vi "flappy--mathstring--load   -- V1.vi"(0 "mathstring IN":string="\"008_040924\" ->   <|  \n\"T\"->  4.0  , \n\"θ\"-> 0 , \n\"vproj\"  -> 0.690,\n\"B\" -> 60 ,\n\"plain\" -> 23\n  |>   , \n  \n    \n\"010_040924\" ->   <|  \n\"T\"->  4.0  , \n\"θ\"-> 30  , \n\"vproj\"  -> 0.600,\n\"B\" -> 60 ,\n\"plain\" -> 23\n  |>   , \n  \n\"011_040924\" ->   <|  \n\"T\"->  4.0  , \n\"θ\"-> 60  , \n\"vproj\"  -> 0.348,\n\"B\" -> 60 ,\n\"plain\" -> 23\n  |>   ,   \n  \n  \n\"002_041024\" ->   <|  \n\"T\"->  4.0  , \n\"θ\"-> 90  , \n\"vproj\"  -> 0.00,\n\"B\" -> 60 ,\n\"plain\" -> 23\n  |>   ,\n   \n    \n\"003_041024\" ->   <|  \n\"T\"->  4.0  , \n\"θ\"-> 120  , \n\"vproj\"  -> -0.340,\n\"B\" -> 60 ,\n\"plain\" -> 23\n  |>   ,\n\n\"004_041024\" ->   <|  \n\"T\"->  4.0  , \n\"θ\"-> 160  , \n\"vproj\"  -> -0.663,\n\"B\" -> 60 ,\n\"plain\" -> 23\n  |>   , \n  \n\"005_041024\" ->   <|  \n\"T\"->  4.0  , \n\"θ\"-> 180  , \n\"vproj\"  -> -0.699,\n\"B\" -> 60 ,\n\"plain\" -> 23\n  |>   , \n  \n\"006_041024\" ->   <|  \n\"T\"->  4.0  , \n\"θ\"-> 165  , \n\"vproj\"  -> -0.677,\n\"B\" -> 60 ,\n\"plain\" -> 23\n  |>   ,\n  \n\"007_041024\" ->   <|  \n\"T\"->  4.0  , \n\"θ\"-> 150  , \n\"vproj\"  -> -0.603,\n\"B\" -> 60 ,\n\"plain\" -> 23\n  |>   ,\n  \n\"008_041024\" ->   <|  \n\"T\"->  4.0  , \n\"θ\"-> 135  , \n\"vproj\"  -> -0.496,\n\"B\" -> 60 ,\n\"plain\" -> 23\n  |>   ,\n  \n\"009_041024\" ->   <|  \n\"T\"->  4.0  , \n\"θ\"-> 105  , \n\"vproj\"  -> -0.178,\n\"B\" -> 60 ,\n\"plain\" -> 23\n  |>   ,\n  \n\"010_041024\" ->   <|  \n\"T\"->  4.0  , \n\"θ\"-> 95  , \n\"vproj\"  -> -0.057,\n\"B\" -> 60 ,\n\"plain\" -> 23\n  |>   ,\n  \n\"011_041024\" ->   <|  \n\"T\"->  4.0  , \n\"θ\"-> 85  , \n\"vproj\"  -> +0.065,\n\"B\" -> 60 ,\n\"plain\" -> 23\n  |>   ,\n  \n\"012_041024\" ->   <|  \n\"T\"->  4.0  , \n\"θ\"-> 75  , \n\"vproj\"  -> +0.183,\n\"B\" -> 60 ,\n\"plain\" -> 23\n  |>   , \n  \n\"013_041024\" ->   <|  \n\"T\"->  4.0  , \n\"θ\"-> 45  , \n\"vproj\"  -> +0.494,\n\"B\" -> 60 ,\n\"plain\" -> 23\n  |>   , \n  \n\"003_041124\" ->   <|  \n\"T\"->  4.0  , \n\"θ\"-> 15  , \n\"vproj\"  -> +0.673,\n\"B\" -> 60 ,\n\"plain\" -> 23\n  |>   ,  \n  \n\"004_041124\" ->   <|  \n\"T\"->  4.0  , \n\"θ\"-> 50  , \n\"vproj\"  -> +0.442,\n\"B\" -> 60 ,\n\"plain\" -> 23\n  |>   ,\n  \n\"005_041124\" ->   <|  \n\"T\"->  4.0  , \n\"θ\"-> 67  , \n\"vproj\"  -> +0.269,\n\"B\" -> 60 ,\n\"plain\" -> 23\n  |>   ,\n  \n\"006_041124\" ->   <|  \n\"T\"->  4.0  , \n\"θ\"-> 55  , \n\"vproj\"  -> +0.397,\n\"B\" -> 60 ,\n\"plain\" -> 23\n  |>   ,   \n  \n\"007_041124\" ->   <|  \n\"T\"->  4.0  , \n\"θ\"-> 112  , \n\"vproj\"  -> -0.260,\n\"B\" -> 60 ,\n\"plain\" -> 23\n  |>   ,  \n  \n\"008_041124\" ->   <|  \n\"T\"->  4.0  , \n\"θ\"-> 128  , \n\"vproj\"  -> -0.432,\n\"B\" -> 60 ,\n\"plain\" -> 23\n  |>   , \n  \n\"009_041124\" ->   <|  \n\"T\"->  4.0  , \n\"θ\"-> 155  , \n\"vproj\"  -> -0.634,\n\"B\" -> 60 ,\n\"plain\" -> 23\n  |>   , \n  \n\"010_041124\" ->   <|  \n\"T\"->  4.0  , \n\"θ\"-> 151  , \n\"vproj\"  -> -0.615,\n\"B\" -> 60 ,\n\"plain\" -> 23\n  |>   ,   \n  \n\"011_041124\" ->   <|  \n\"T\"->  4.0  , \n\"θ\"-> 157  , \n\"vproj\"  -> -0.648,\n\"B\" -> 60 ,\n\"plain\" -> 23\n  |>   ,  \n  \n  \n\"002_041224\" ->   <|  \n\"T\"->  4.0  , \n\"θ\"-> 170  , \n\"vproj\"  -> -0.690,\n\"B\" -> 60 ,\n\"plain\" -> 23\n  |>   ,\n  \n\"003_041224\" ->   <|  \n\"T\"->  4.0  , \n\"θ\"-> 153  , \n\"vproj\"  -> -0.625,\n\"B\" -> 60 ,\n\"plain\" -> 23\n  |>   , \n  \n  \n\"004_041224\" ->   <|  \n\"T\"->  10.0  , \n\"θ\"-> 153  , \n\"vproj\"  -> -0.625,\n\"B\" -> 60 ,\n\"plain\" -> 23\n  |>   ,\n  \n  \n\"005_041224\" ->   <|  \n\"T\"->  20.0  , \n\"θ\"-> 153  , \n\"vproj\"  -> -0.625,\n\"B\" -> 60 ,\n\"plain\" -> 23\n  |>   , \n  \n\"006_041224\" ->   <|  \n\"T\"->  30.0  , \n\"θ\"-> 153  , \n\"vproj\"  -> -0.625,\n\"B\" -> 60 ,\n\"plain\" -> 23\n  |>   ,\n  \n  \n\"007_041224\" ->   <|  \n\"T\"->  25.0  , \n\"θ\"-> 153  , \n\"vproj\"  -> -0.625,\n\"B\" -> 60 ,\n\"plain\" -> 23\n  |>   , \n  \n  \n\"008_041224\" ->   <|  \n\"T\"->  15.0  , \n\"θ\"-> 153  , \n\"vproj\"  -> -0.625,\n\"B\" -> 60 ,\n\"plain\" -> 23\n  |>   , \n  \n  \n\"009_041224\" ->   <|  \n\"T\"->  17.0  , \n\"θ\"-> 153  , \n\"vproj\"  -> -0.625,\n\"B\" -> 60 ,\n\"plain\" -> 23\n  |>   , \n  \n  \n  \n  \n\"004_042224\" ->   <|  \n\"T\"->  4.0  , \n\"θ\"-> 15  , \n\"vproj\"  -> +0.670,\n\"B\" -> 60 ,\n\"plain\" -> 23\n  |>   ,   \n  \n  \n\"005_042224\" ->   <|  \n\"T\"->  4.0  , \n\"θ\"-> 20  , \n\"vproj\"  -> +0.651,\n\"B\" -> 60 ,\n\"plain\" -> 23\n  |>   ,\n  \n\"006_042224\" ->   <|  \n\"T\"->  4.0  , \n\"θ\"-> 25  , \n\"vproj\"  -> +0.628,\n\"B\" -> 60 ,\n\"plain\" -> 23\n  |>   ,\n  \n  \n\"007_042224\" ->   <|  \n\"T\"->  4.0  , \n\"θ\"-> 30  , \n\"vproj\"  -> +0.603,\n\"B\" -> 60 ,\n\"plain\" -> 23\n  |>   , \n  \n\"008_042224\" ->   <|  \n\"T\"->  4.0  , \n\"θ\"-> 40  , \n\"vproj\"  -> +0.533,\n\"B\" -> 60 ,\n\"plain\" -> 23\n  |>   ,\n  \n  \n  \n\"009_042224\" ->   <|  \n\"T\"->  4.0  , \n\"θ\"-> 53  , \n\"vproj\"  -> +0.415,\n\"B\" -> 60 ,\n\"plain\" -> 23\n  |>   , \n  \n  \n\"010_042224\" ->   <|  \n\"T\"->  4.0  , \n\"θ\"-> 65  , \n\"vproj\"  -> +0.288,\n\"B\" -> 60 ,\n\"plain\" -> 23\n  |>   ,   \n  \n  \n\"011_042224\" ->   <|  \n\"T\"->  4.0  , \n\"θ\"-> 160  , \n\"vproj\"  -> -0.661,\n\"B\" -> 60 ,\n\"plain\" -> 23\n  |>   ,  \n  \n  \n\"013_042224\" ->   <|  \n\"T\"->  4.0  , \n\"θ\"-> 163  , \n\"vproj\"  -> -0.674,\n\"B\" -> 60 ,\n\"plain\" -> 23\n  |>   ,                                                               \n                                              ", 2 "MAIN folder":path=path "/Users/arkadyshekhter/Library/CloudStorage/Dropbox/shared_KimValBra/UTe2--Apr2024", 9 "data file parameters map":map{T2, T3}(c390), 11 "what? IN":T1={"ignore set of !"=TRUE, "set (1T|2B)"=0, "ignore θ !"=FALSE, "ignore B !"=FALSE, "T (K)"=1.0, "ignore T !"=TRUE, "θ (∘)"=0.0, "B (T)"=0.0, "lookup"={"set of lookup"={0=1.0, 1=2.0}, "all set of"={1.0, 2.0}, "T lookup"={0=0.12, 1=0.122, 2=0.14, 3=0.148, 4=0.15, 5=0.157, 6=0.16, 7=0.168, 8=0.17, 9=0.178, 10=0.179, 11=0.18, 12=0.19, 13=0.197, 14=0.2, 15=0.249, 16=0.25, 17=0.255, 18=0.26, 19=0.3, 20=0.307, 21=0.308, 22=0.31, 23=0.36, 24=0.42, 25=0.43, 26=0.438, 27=0.512, 28=0.52, 29=0.53, 30=0.61, 31=0.62, 32=0.63, 33=0.677, 34=0.81, 35=0.82, 36=0.83, 37=1.0, 38=1.1, 39=1.12, 40=1.13, 41=1.25, 42=1.28, 43=1.31, 44=1.39, 45=1.5, 46=1.52, 47=1.55, 48=1.6, 49=1.7, 50=1.8, 51=1.9, 52=2.1, 53=2.3, 54=3.0, 55=3.07, 56=3.1, 57=3.11, 58=5.5, 59=5.7, 60=5.75}, "θ lookup"={0=0.0, 1=30.0, 2=45.0, 3=60.0, 4=90.0}, "B lookup"={0=0.0, 1=1.0, 2=2.0, 3=4.0, 4=5.0, 5=6.0, 6=7.0, 7=8.0, 8=9.0, 9=10.0, 10=11.0, 11=12.0}, "all T's"={0.12, 0.122, 0.14, 0.148, 0.15, 0.157, 0.16, 0.168, 0.17, 0.178, 0.179, 0.18, 0.19, 0.197, 0.2, 0.249, 0.25, 0.255, 0.26, 0.3, 0.307, 0.308, 0.31, 0.36, 0.42, 0.43, 0.438, 0.512, 0.52, 0.53, 0.61, 0.62, 0.63, 0.677, 0.81, 0.82, 0.83, 1.0, 1.1, 1.12, 1.13, 1.25, 1.28, 1.31, 1.39, 1.5, 1.52, 1.55, 1.6, 1.7, 1.8, 1.9, 2.1, 2.3, 3.0, 3.07, 3.1, 3.11, 5.5, 5.7, 5.75}, "all θ's"={0.0, 30.0, 45.0, 60.0, 90.0}, "all B's"={0.0, 1.0, 2.0, 4.0, 5.0, 6.0, 7.0, 8.0, 9.0, 10.0, 11.0, 12.0}, "all sides"={4000.0, 8000.0}, "side lookup"={0=4000.0, 1=8000.0}}} {"B (T)" items=["0.000", "1.000", "2.000", "4.000", "5.000", "6.000", "7.000", "8.000", "9.000", "10.000", "11.000", "12.000"]; "θ (∘)" items=["0.000", "30.000", "45.000", "60.000", "90.000"]; "T (K)" items=["0.120", "0.122", "0.140", "0.148", "0.150", "0.157", "0.160", "0.168", "0.170", "0.178", "0.179", "0.180", "0.190", "0.197", "0.200", "0.249", "0.250", "0.255", "0.260", "0.300", "0.307", "0.308", "0.310", "0.360", "0.420", "0.430", "0.438", "0.512", "0.520", "0.530", "0.610", "0.620", "0.630", "0.677", "0.810", "0.820", "0.830", "1.000", "1.100", "1.120", "1.130", "1.250", "1.280", "1.310", "1.390", "1.500", "1.520", "1.550", "1.600", "1.700", "1.800", "1.900", "2.100", "2.300", "3.000", "3.070", "3.100", "3.110", "5.500", "5.700", "5.750"]; "set (1T|2B)" items=["1", "2"]}, 13 "data file pattern":string="p_c3_*.tdms") -> (4 "all short filenames":map{string, string}(c390), 6 "temps&degs":map{string, map{T2, dbl}}(c390), 8 "mathematica thing":map{string, map{T2, dbl}}(c390)={"002_041024"={enum."ζ"=0.0, enum."τ1"=0.0, enum."τS"=0.0, enum."τN"=0.0, enum."τC"=0.0, enum."κ0"=0.0, enum."m1"=0.0, enum."m2"=0.0, enum."m3"=0.0, enum."T (K)"=4.0, enum."B (T)"=60.0, enum."θ (deg)"=90.0, enum."Re(offset)"=0.0, enum."Im(offset)"=0.0, enum."στ1"=0.0, enum."στS"=0.0, enum."στN"=0.0, enum."τ11"=0.0, enum."τ12"=0.0, enum."τ22"=0.0, enum."τN1"=0.0, enum."τN2"=0.0, enum."σηlogτ1"=0.0, enum."σηlogτS"=0.0, enum."σηlogτN"=0.0, enum."σlogτ1"=0.0, enum."σlogτS"=0.0, enum."σlogτN"=0.0, enum."σητ1"=0.0, enum."σητS"=0.0, enum."σητN"=0.0, enum."noiseT"=0.0, enum."plain"=23.0, enum."vproj"=0.0}, "002_041224"={enum."ζ"=0.0, enum."τ1"=0.0, enum."τS"=0.0, enum."τN"=0.0, enum."τC"=0.0, enum."κ0"=0.0, enum."m1"=0.0, enum."m2"=0.0, enum."m3"=0.0, enum."T (K)"=4.0, enum."B (T)"=60.0, enum."θ (deg)"=170.0, enum."Re(offset)"=0.0, enum."Im(offset)"=0.0, enum."στ1"=0.0, enum."στS"=0.0, enum."στN"=0.0, enum."τ11"=0.0, enum."τ12"=0.0, enum."τ22"=0.0, enum."τN1"=0.0, enum."τN2"=0.0, enum."σηlogτ1"=0.0, enum."σηlogτS"=0.0, enum."σηlogτN"=0.0, enum."σlogτ1"=0.0, enum."σlogτS"=0.0, enum."σlogτN"=0.0, enum."σητ1"=0.0, enum."σητS"=0.0, enum."σητN"=0.0, enum."noiseT"=0.0, enum."plain"=23.0, enum."vproj"=-0.69}, "003_041024"={enum."ζ"=0.0, enum."τ1"=0.0, enum."τS"=0.0, enum."τN"=0.0, enum."τC"=0.0, enum."κ0"=0.0, enum."m1"=0.0, enum."m2"=0.0, enum."m3"=0.0, enum."T (K)"=4.0, enum."B (T)"=60.0, enum."θ (deg)"=120.0, enum."Re(offset)"=0.0, enum."Im(offset)"=0.0, enum."στ1"=0.0, enum."στS"=0.0, enum."στN"=0.0, enum."τ11"=0.0, enum."τ12"=0.0, enum."τ22"=0.0, enum."τN1"=0.0, enum."τN2"=0.0, enum."σηlogτ1"=0.0, enum."σηlogτS"=0.0, enum."σηlogτN"=0.0, enum."σlogτ1"=0.0, enum."σlogτS"=0.0, enum."σlogτN"=0.0, enum."σητ1"=0.0, enum."σητS"=0.0, enum."σητN"=0.0, enum."noiseT"=0.0, enum."plain"=23.0, enum."vproj"=-0.34}, "003_041124"={enum."ζ"=0.0, enum."τ1"=0.0, enum."τS"=0.0, enum."τN"=0.0, enum."τC"=0.0, enum."κ0"=0.0, enum."m1"=0.0, enum."m2"=0.0, enum."m3"=0.0, enum."T (K)"=4.0, enum."B (T)"=60.0, enum."θ (deg)"=15.0, enum."Re(offset)"=0.0, enum."Im(offset)"=0.0, enum."στ1"=0.0, enum."στS"=0.0, enum."στN"=0.0, enum."τ11"=0.0, enum."τ12"=0.0, enum."τ22"=0.0, enum."τN1"=0.0, enum."τN2"=0.0, enum."σηlogτ1"=0.0, enum."σηlogτS"=0.0, enum."σηlogτN"=0.0, enum."σlogτ1"=0.0, enum."σlogτS"=0.0, enum."σlogτN"=0.0, enum."σητ1"=0.0, enum."σητS"=0.0, enum."σητN"=0.0, enum."noiseT"=0.0, enum."plain"=23.0, enum."vproj"=0.673}, "003_041224"={enum."ζ"=0.0, enum."τ1"=0.0, enum."τS"=0.0, enum."τN"=0.0, enum."τC"=0.0, enum."κ0"=0.0, enum."m1"=0.0, enum."m2"=0.0, enum."m3"=0.0, enum."T (K)"=4.0, enum."B (T)"=60.0, enum."θ (deg)"=153.0, enum."Re(offset)"=0.0, enum."Im(offset)"=0.0, enum."στ1"=0.0, enum."στS"=0.0, enum."στN"=0.0, enum."τ11"=0.0, enum."τ12"=0.0, enum."τ22"=0.0, enum."τN1"=0.0, enum."τN2"=0.0, enum."σηlogτ1"=0.0, enum."σηlogτS"=0.0, enum."σηlogτN"=0.0, enum."σlogτ1"=0.0, enum."σlogτS"=0.0, enum."σlogτN"=0.0, enum."σητ1"=0.0, enum."σητS"=0.0, enum."σητN"=0.0, enum."noiseT"=0.0, enum."plain"=23.0, enum."vproj"=-0.625}, "004_041024"={enum."ζ"=0.0, enum."τ1"=0.0, enum."τS"=0.0, enum."τN"=0.0, enum."τC"=0.0, enum."κ0"=0.0, enum."m1"=0.0, enum."m2"=0.0, enum."m3"=0.0, enum."T (K)"=4.0, enum."B (T)"=60.0, enum."θ (deg)"=160.0, enum."Re(offset)"=0.0, enum."Im(offset)"=0.0, enum."στ1"=0.0, enum."στS"=0.0, enum."στN"=0.0, enum."τ11"=0.0, enum."τ12"=0.0, enum."τ22"=0.0, enum."τN1"=0.0, enum."τN2"=0.0, enum."σηlogτ1"=0.0, enum."σηlogτS"=0.0, enum."σηlogτN"=0.0, enum."σlogτ1"=0.0, enum."σlogτS"=0.0, enum."σlogτN"=0.0, enum."σητ1"=0.0, enum."σητS"=0.0, enum."σητN"=0.0, enum."noiseT"=0.0, enum."plain"=23.0, enum."vproj"=-0.663}, "004_041124"={enum."ζ"=0.0, enum."τ1"=0.0, enum."τS"=0.0, enum."τN"=0.0, enum."τC"=0.0, enum."κ0"=0.0, enum."m1"=0.0, enum."m2"=0.0, enum."m3"=0.0, enum."T (K)"=4.0, enum."B (T)"=60.0, enum."θ (deg)"=50.0, enum."Re(offset)"=0.0, enum."Im(offset)"=0.0, enum."στ1"=0.0, enum."στS"=0.0, enum."στN"=0.0, enum."τ11"=0.0, enum."τ12"=0.0, enum."τ22"=0.0, enum."τN1"=0.0, enum."τN2"=0.0, enum."σηlogτ1"=0.0, enum."σηlogτS"=0.0, enum."σηlogτN"=0.0, enum."σlogτ1"=0.0, enum."σlogτS"=0.0, enum."σlogτN"=0.0, enum."σητ1"=0.0, enum."σητS"=0.0, enum."σητN"=0.0, enum."noiseT"=0.0, enum."plain"=23.0, enum."vproj"=0.442}, "004_041224"={enum."ζ"=0.0, enum."τ1"=0.0, enum."τS"=0.0, enum."τN"=0.0, enum."τC"=0.0, enum."κ0"=0.0, enum."m1"=0.0, enum."m2"=0.0, enum."m3"=0.0, enum."T (K)"=10.0, enum."B (T)"=60.0, enum."θ (deg)"=153.0, enum."Re(offset)"=0.0, enum."Im(offset)"=0.0, enum."στ1"=0.0, enum."στS"=0.0, enum."στN"=0.0, enum."τ11"=0.0, enum."τ12"=0.0, enum."τ22"=0.0, enum."τN1"=0.0, enum."τN2"=0.0, enum."σηlogτ1"=0.0, enum."σηlogτS"=0.0, enum."σηlogτN"=0.0, enum."σlogτ1"=0.0, enum."σlogτS"=0.0, enum."σlogτN"=0.0, enum."σητ1"=0.0, enum."σητS"=0.0, enum."σητN"=0.0, enum."noiseT"=0.0, enum."plain"=23.0, enum."vproj"=-0.625}, "004_042224"={enum."ζ"=0.0, enum."τ1"=0.0, enum."τS"=0.0, enum."τN"=0.0, enum."τC"=0.0, enum."κ0"=0.0, enum."m1"=0.0, enum."m2"=0.0, enum."m3"=0.0, enum."T (K)"=4.0, enum."B (T)"=60.0, enum."θ (deg)"=15.0, enum."Re(offset)"=0.0, enum."Im(offset)"=0.0, enum."στ1"=0.0, enum."στS"=0.0, enum."στN"=0.0, enum."τ11"=0.0, enum."τ12"=0.0, enum."τ22"=0.0, enum."τN1"=0.0, enum."τN2"=0.0, enum."σηlogτ1"=0.0, enum."σηlogτS"=0.0, enum."σηlogτN"=0.0, enum."σlogτ1"=0.0, enum."σlogτS"=0.0, enum."σlogτN"=0.0, enum."σητ1"=0.0, enum."σητS"=0.0, enum."σητN"=0.0, enum."noiseT"=0.0, enum."plain"=23.0, enum."vproj"=0.67}, "005_041024"={enum."ζ"=0.0, enum."τ1"=0.0, enum."τS"=0.0, enum."τN"=0.0, enum."τC"=0.0, enum."κ0"=0.0, enum."m1"=0.0, enum."m2"=0.0, enum."m3"=0.0, enum."T (K)"=4.0, enum."B (T)"=60.0, enum."θ (deg)"=180.0, enum."Re(offset)"=0.0, enum."Im(offset)"=0.0, enum."στ1"=0.0, enum."στS"=0.0, enum."στN"=0.0, enum."τ11"=0.0, enum."τ12"=0.0, enum."τ22"=0.0, enum."τN1"=0.0, enum."τN2"=0.0, enum."σηlogτ1"=0.0, enum."σηlogτS"=0.0, enum."σηlogτN"=0.0, enum."σlogτ1"=0.0, enum."σlogτS"=0.0, enum."σlogτN"=0.0, enum."σητ1"=0.0, enum."σητS"=0.0, enum."σητN"=0.0, enum."noiseT"=0.0, enum."plain"=23.0, enum."vproj"=-0.699}, "005_041124"={enum."ζ"=0.0, enum."τ1"=0.0, enum."τS"=0.0, enum."τN"=0.0, enum."τC"=0.0, enum."κ0"=0.0, enum."m1"=0.0, enum."m2"=0.0, enum."m3"=0.0, enum."T (K)"=4.0, enum."B (T)"=60.0, enum."θ (deg)"=67.0, enum."Re(offset)"=0.0, enum."Im(offset)"=0.0, enum."στ1"=0.0, enum."στS"=0.0, enum."στN"=0.0, enum."τ11"=0.0, enum."τ12"=0.0, enum."τ22"=0.0, enum."τN1"=0.0, enum."τN2"=0.0, enum."σηlogτ1"=0.0, enum."σηlogτS"=0.0, enum."σηlogτN"=0.0, enum."σlogτ1"=0.0, enum."σlogτS"=0.0, enum."σlogτN"=0.0, enum."σητ1"=0.0, enum."σητS"=0.0, enum."σητN"=0.0, enum."noiseT"=0.0, enum."plain"=23.0, enum."vproj"=0.269}, "005_041224"={enum."ζ"=0.0, enum."τ1"=0.0, enum."τS"=0.0, enum."τN"=0.0, enum."τC"=0.0, enum."κ0"=0.0, enum."m1"=0.0, enum."m2"=0.0, enum."m3"=0.0, enum."T (K)"=20.0, enum."B (T)"=60.0, enum."θ (deg)"=153.0, enum."Re(offset)"=0.0, enum."Im(offset)"=0.0, enum."στ1"=0.0, enum."στS"=0.0, enum."στN"=0.0, enum."τ11"=0.0, enum."τ12"=0.0, enum."τ22"=0.0, enum."τN1"=0.0, enum."τN2"=0.0, enum."σηlogτ1"=0.0, enum."σηlogτS"=0.0, enum."σηlogτN"=0.0, enum."σlogτ1"=0.0, enum."σlogτS"=0.0, enum."σlogτN"=0.0, enum."σητ1"=0.0, enum."σητS"=0.0, enum."σητN"=0.0, enum."noiseT"=0.0, enum."plain"=23.0, enum."vproj"=-0.625}, "005_042224"={enum."ζ"=0.0, enum."τ1"=0.0, enum."τS"=0.0, enum."τN"=0.0, enum."τC"=0.0, enum."κ0"=0.0, enum."m1"=0.0, enum."m2"=0.0, enum."m3"=0.0, enum."T (K)"=4.0, enum."B (T)"=60.0, enum."θ (deg)"=20.0, enum."Re(offset)"=0.0, enum."Im(offset)"=0.0, enum."στ1"=0.0, enum."στS"=0.0, enum."στN"=0.0, enum."τ11"=0.0, enum."τ12"=0.0, enum."τ22"=0.0, enum."τN1"=0.0, enum."τN2"=0.0, enum."σηlogτ1"=0.0, enum."σηlogτS"=0.0, enum."σηlogτN"=0.0, enum."σlogτ1"=0.0, enum."σlogτS"=0.0, enum."σlogτN"=0.0, enum."σητ1"=0.0, enum."σητS"=0.0, enum."σητN"=0.0, enum."noiseT"=0.0, enum."plain"=23.0, enum."vproj"=0.651}, "006_041024"={enum."ζ"=0.0, enum."τ1"=0.0, enum."τS"=0.0, enum."τN"=0.0, enum."τC"=0.0, enum."κ0"=0.0, enum."m1"=0.0, enum."m2"=0.0, enum."m3"=0.0, enum."T (K)"=4.0, enum."B (T)"=60.0, enum."θ (deg)"=165.0, enum."Re(offset)"=0.0, enum."Im(offset)"=0.0, enum."στ1"=0.0, enum."στS"=0.0, enum."στN"=0.0, enum."τ11"=0.0, enum."τ12"=0.0, enum."τ22"=0.0, enum."τN1"=0.0, enum."τN2"=0.0, enum."σηlogτ1"=0.0, enum."σηlogτS"=0.0, enum."σηlogτN"=0.0, enum."σlogτ1"=0.0, enum."σlogτS"=0.0, enum."σlogτN"=0.0, enum."σητ1"=0.0, enum."σητS"=0.0, enum."σητN"=0.0, enum."noiseT"=0.0, enum."plain"=23.0, enum."vproj"=-0.677}, "006_041124"={enum."ζ"=0.0, enum."τ1"=0.0, enum."τS"=0.0, enum."τN"=0.0, enum."τC"=0.0, enum."κ0"=0.0, enum."m1"=0.0, enum."m2"=0.0, enum."m3"=0.0, enum."T (K)"=4.0, enum."B (T)"=60.0, enum."θ (deg)"=55.0, enum."Re(offset)"=0.0, enum."Im(offset)"=0.0, enum."στ1"=0.0, enum."στS"=0.0, enum."στN"=0.0, enum."τ11"=0.0, enum."τ12"=0.0, enum."τ22"=0.0, enum."τN1"=0.0, enum."τN2"=0.0, enum."σηlogτ1"=0.0, enum."σηlogτS"=0.0, enum."σηlogτN"=0.0, enum."σlogτ1"=0.0, enum."σlogτS"=0.0, enum."σlogτN"=0.0, enum."σητ1"=0.0, enum."σητS"=0.0, enum."σητN"=0.0, enum."noiseT"=0.0, enum."plain"=23.0, enum."vproj"=0.397}, "006_041224"={enum."ζ"=0.0, enum."τ1"=0.0, enum."τS"=0.0, enum."τN"=0.0, enum."τC"=0.0, enum."κ0"=0.0, enum."m1"=0.0, enum."m2"=0.0, enum."m3"=0.0, enum."T (K)"=30.0, enum."B (T)"=60.0, enum."θ (deg)"=153.0, enum."Re(offset)"=0.0, enum."Im(offset)"=0.0, enum."στ1"=0.0, enum."στS"=0.0, enum."στN"=0.0, enum."τ11"=0.0, enum."τ12"=0.0, enum."τ22"=0.0, enum."τN1"=0.0, enum."τN2"=0.0, enum."σηlogτ1"=0.0, enum."σηlogτS"=0.0, enum."σηlogτN"=0.0, enum."σlogτ1"=0.0, enum."σlogτS"=0.0, enum."σlogτN"=0.0, enum."σητ1"=0.0, enum."σητS"=0.0, enum."σητN"=0.0, enum."noiseT"=0.0, enum."plain"=23.0, enum."vproj"=-0.625}, "006_042224"={enum."ζ"=0.0, enum."τ1"=0.0, enum."τS"=0.0, enum."τN"=0.0, enum."τC"=0.0, enum."κ0"=0.0, enum."m1"=0.0, enum."m2"=0.0, enum."m3"=0.0, enum."T (K)"=4.0, enum."B (T)"=60.0, enum."θ (deg)"=25.0, enum."Re(offset)"=0.0, enum."Im(offset)"=0.0, enum."στ1"=0.0, enum."στS"=0.0, enum."στN"=0.0, enum."τ11"=0.0, enum."τ12"=0.0, enum."τ22"=0.0, enum."τN1"=0.0, enum."τN2"=0.0, enum."σηlogτ1"=0.0, enum."σηlogτS"=0.0, enum."σηlogτN"=0.0, enum."σlogτ1"=0.0, enum."σlogτS"=0.0, enum."σlogτN"=0.0, enum."σητ1"=0.0, enum."σητS"=0.0, enum."σητN"=0.0, enum."noiseT"=0.0, enum."plain"=23.0, enum."vproj"=0.628}, "007_041024"={enum."ζ"=0.0, enum."τ1"=0.0, enum."τS"=0.0, enum."τN"=0.0, enum."τC"=0.0, enum."κ0"=0.0, enum."m1"=0.0, enum."m2"=0.0, enum."m3"=0.0, enum."T (K)"=4.0, enum."B (T)"=60.0, enum."θ (deg)"=150.0, enum."Re(offset)"=0.0, enum."Im(offset)"=0.0, enum."στ1"=0.0, enum."στS"=0.0, enum."στN"=0.0, enum."τ11"=0.0, enum."τ12"=0.0, enum."τ22"=0.0, enum."τN1"=0.0, enum."τN2"=0.0, enum."σηlogτ1"=0.0, enum."σηlogτS"=0.0, enum."σηlogτN"=0.0, enum."σlogτ1"=0.0, enum."σlogτS"=0.0, enum."σlogτN"=0.0, enum."σητ1"=0.0, enum."σητS"=0.0, enum."σητN"=0.0, enum."noiseT"=0.0, enum."plain"=23.0, enum."vproj"=-0.603}, "007_041124"={enum."ζ"=0.0, enum."τ1"=0.0, enum."τS"=0.0, enum."τN"=0.0, enum."τC"=0.0, enum."κ0"=0.0, enum."m1"=0.0, enum."m2"=0.0, enum."m3"=0.0, enum."T (K)"=4.0, enum."B (T)"=60.0, enum."θ (deg)"=112.0, enum."Re(offset)"=0.0, enum."Im(offset)"=0.0, enum."στ1"=0.0, enum."στS"=0.0, enum."στN"=0.0, enum."τ11"=0.0, enum."τ12"=0.0, enum."τ22"=0.0, enum."τN1"=0.0, enum."τN2"=0.0, enum."σηlogτ1"=0.0, enum."σηlogτS"=0.0, enum."σηlogτN"=0.0, enum."σlogτ1"=0.0, enum."σlogτS"=0.0, enum."σlogτN"=0.0, enum."σητ1"=0.0, enum."σητS"=0.0, enum."σητN"=0.0, enum."noiseT"=0.0, enum."plain"=23.0, enum."vproj"=-0.26}, "007_041224"={enum."ζ"=0.0, enum."τ1"=0.0, enum."τS"=0.0, enum."τN"=0.0, enum."τC"=0.0, enum."κ0"=0.0, enum."m1"=0.0, enum."m2"=0.0, enum."m3"=0.0, enum."T (K)"=25.0, enum."B (T)"=60.0, enum."θ (deg)"=153.0, enum."Re(offset)"=0.0, enum."Im(offset)"=0.0, enum."στ1"=0.0, enum."στS"=0.0, enum."στN"=0.0, enum."τ11"=0.0, enum."τ12"=0.0, enum."τ22"=0.0, enum."τN1"=0.0, enum."τN2"=0.0, enum."σηlogτ1"=0.0, enum."σηlogτS"=0.0, enum."σηlogτN"=0.0, enum."σlogτ1"=0.0, enum."σlogτS"=0.0, enum."σlogτN"=0.0, enum."σητ1"=0.0, enum."σητS"=0.0, enum."σητN"=0.0, enum."noiseT"=0.0, enum."plain"=23.0, enum."vproj"=-0.625}, "007_042224"={enum."ζ"=0.0, enum."τ1"=0.0, enum."τS"=0.0, enum."τN"=0.0, enum."τC"=0.0, enum."κ0"=0.0, enum."m1"=0.0, enum."m2"=0.0, enum."m3"=0.0, enum."T (K)"=4.0, enum."B (T)"=60.0, enum."θ (deg)"=30.0, enum."Re(offset)"=0.0, enum."Im(offset)"=0.0, enum."στ1"=0.0, enum."στS"=0.0, enum."στN"=0.0, enum."τ11"=0.0, enum."τ12"=0.0, enum."τ22"=0.0, enum."τN1"=0.0, enum."τN2"=0.0, enum."σηlogτ1"=0.0, enum."σηlogτS"=0.0, enum."σηlogτN"=0.0, enum."σlogτ1"=0.0, enum."σlogτS"=0.0, enum."σlogτN"=0.0, enum."σητ1"=0.0, enum."σητS"=0.0, enum."σητN"=0.0, enum."noiseT"=0.0, enum."plain"=23.0, enum."vproj"=0.603}, "008_040924"={enum."ζ"=0.0, enum."τ1"=0.0, enum."τS"=0.0, enum."τN"=0.0, enum."τC"=0.0, enum."κ0"=0.0, enum."m1"=0.0, enum."m2"=0.0, enum."m3"=0.0, enum."T (K)"=4.0, enum."B (T)"=60.0, enum."θ (deg)"=0.0, enum."Re(offset)"=0.0, enum."Im(offset)"=0.0, enum."στ1"=0.0, enum."στS"=0.0, enum."στN"=0.0, enum."τ11"=0.0, enum."τ12"=0.0, enum."τ22"=0.0, enum."τN1"=0.0, enum."τN2"=0.0, enum."σηlogτ1"=0.0, enum."σηlogτS"=0.0, enum."σηlogτN"=0.0, enum."σlogτ1"=0.0, enum."σlogτS"=0.0, enum."σlogτN"=0.0, enum."σητ1"=0.0, enum."σητS"=0.0, enum."σητN"=0.0, enum."noiseT"=0.0, enum."plain"=23.0, enum."vproj"=0.69}, "008_041024"={enum."ζ"=0.0, enum."τ1"=0.0, enum."τS"=0.0, enum."τN"=0.0, enum."τC"=0.0, enum."κ0"=0.0, enum."m1"=0.0, enum."m2"=0.0, enum."m3"=0.0, enum."T (K)"=4.0, enum."B (T)"=60.0, enum."θ (deg)"=135.0, enum."Re(offset)"=0.0, enum."Im(offset)"=0.0, enum."στ1"=0.0, enum."στS"=0.0, enum."στN"=0.0, enum."τ11"=0.0, enum."τ12"=0.0, enum."τ22"=0.0, enum."τN1"=0.0, enum."τN2"=0.0, enum."σηlogτ1"=0.0, enum."σηlogτS"=0.0, enum."σηlogτN"=0.0, enum."σlogτ1"=0.0, enum."σlogτS"=0.0, enum."σlogτN"=0.0, enum."σητ1"=0.0, enum."σητS"=0.0, enum."σητN"=0.0, enum."noiseT"=0.0, enum."plain"=23.0, enum."vproj"=-0.496}, "008_041124"={enum."ζ"=0.0, enum."τ1"=0.0, enum."τS"=0.0, enum."τN"=0.0, enum."τC"=0.0, enum."κ0"=0.0, enum."m1"=0.0, enum."m2"=0.0, enum."m3"=0.0, enum."T (K)"=4.0, enum."B (T)"=60.0, enum."θ (deg)"=128.0, enum."Re(offset)"=0.0, enum."Im(offset)"=0.0, enum."στ1"=0.0, enum."στS"=0.0, enum."στN"=0.0, enum."τ11"=0.0, enum."τ12"=0.0, enum."τ22"=0.0, enum."τN1"=0.0, enum."τN2"=0.0, enum."σηlogτ1"=0.0, enum."σηlogτS"=0.0, enum."σηlogτN"=0.0, enum."σlogτ1"=0.0, enum."σlogτS"=0.0, enum."σlogτN"=0.0, enum."σητ1"=0.0, enum."σητS"=0.0, enum."σητN"=0.0, enum."noiseT"=0.0, enum."plain"=23.0, enum."vproj"=-0.432}, "008_041224"={enum."ζ"=0.0, enum."τ1"=0.0, enum."τS"=0.0, enum."τN"=0.0, enum."τC"=0.0, enum."κ0"=0.0, enum."m1"=0.0, enum."m2"=0.0, enum."m3"=0.0, enum."T (K)"=15.0, enum."B (T)"=60.0, enum."θ (deg)"=153.0, enum."Re(offset)"=0.0, enum."Im(offset)"=0.0, enum."στ1"=0.0, enum."στS"=0.0, enum."στN"=0.0, enum."τ11"=0.0, enum."τ12"=0.0, enum."τ22"=0.0, enum."τN1"=0.0, enum."τN2"=0.0, enum."σηlogτ1"=0.0, enum."σηlogτS"=0.0, enum."σηlogτN"=0.0, enum."σlogτ1"=0.0, enum."σlogτS"=0.0, enum."σlogτN"=0.0, enum."σητ1"=0.0, enum."σητS"=0.0, enum."σητN"=0.0, enum."noiseT"=0.0, enum."plain"=23.0, enum."vproj"=-0.625}, "008_042224"={enum."ζ"=0.0, enum."τ1"=0.0, enum."τS"=0.0, enum."τN"=0.0, enum."τC"=0.0, enum."κ0"=0.0, enum."m1"=0.0, enum."m2"=0.0, enum."m3"=0.0, enum."T (K)"=4.0, enum."B (T)"=60.0, enum."θ (deg)"=40.0, enum."Re(offset)"=0.0, enum."Im(offset)"=0.0, enum."στ1"=0.0, enum."στS"=0.0, enum."στN"=0.0, enum."τ11"=0.0, enum."τ12"=0.0, enum."τ22"=0.0, enum."τN1"=0.0, enum."τN2"=0.0, enum."σηlogτ1"=0.0, enum."σηlogτS"=0.0, enum."σηlogτN"=0.0, enum."σlogτ1"=0.0, enum."σlogτS"=0.0, enum."σlogτN"=0.0, enum."σητ1"=0.0, enum."σητS"=0.0, enum."σητN"=0.0, enum."noiseT"=0.0, enum."plain"=23.0, enum."vproj"=0.533}, "009_041024"={enum."ζ"=0.0, enum."τ1"=0.0, enum."τS"=0.0, enum."τN"=0.0, enum."τC"=0.0, enum."κ0"=0.0, enum."m1"=0.0, enum."m2"=0.0, enum."m3"=0.0, enum."T (K)"=4.0, enum."B (T)"=60.0, enum."θ (deg)"=105.0, enum."Re(offset)"=0.0, enum."Im(offset)"=0.0, enum."στ1"=0.0, enum."στS"=0.0, enum."στN"=0.0, enum."τ11"=0.0, enum."τ12"=0.0, enum."τ22"=0.0, enum."τN1"=0.0, enum."τN2"=0.0, enum."σηlogτ1"=0.0, enum."σηlogτS"=0.0, enum."σηlogτN"=0.0, enum."σlogτ1"=0.0, enum."σlogτS"=0.0, enum."σlogτN"=0.0, enum."σητ1"=0.0, enum."σητS"=0.0, enum."σητN"=0.0, enum."noiseT"=0.0, enum."plain"=23.0, enum."vproj"=-0.178}, "009_041124"={enum."ζ"=0.0, enum."τ1"=0.0, enum."τS"=0.0, enum."τN"=0.0, enum."τC"=0.0, enum."κ0"=0.0, enum."m1"=0.0, enum."m2"=0.0, enum."m3"=0.0, enum."T (K)"=4.0, enum."B (T)"=60.0, enum."θ (deg)"=155.0, enum."Re(offset)"=0.0, enum."Im(offset)"=0.0, enum."στ1"=0.0, enum."στS"=0.0, enum."στN"=0.0, enum."τ11"=0.0, enum."τ12"=0.0, enum."τ22"=0.0, enum."τN1"=0.0, enum."τN2"=0.0, enum."σηlogτ1"=0.0, enum."σηlogτS"=0.0, enum."σηlogτN"=0.0, enum."σlogτ1"=0.0, enum."σlogτS"=0.0, enum."σlogτN"=0.0, enum."σητ1"=0.0, enum."σητS"=0.0, enum."σητN"=0.0, enum."noiseT"=0.0, enum."plain"=23.0, enum."vproj"=-0.634}, "009_041224"={enum."ζ"=0.0, enum."τ1"=0.0, enum."τS"=0.0, enum."τN"=0.0, enum."τC"=0.0, enum."κ0"=0.0, enum."m1"=0.0, enum."m2"=0.0, enum."m3"=0.0, enum."T (K)"=17.0, enum."B (T)"=60.0, enum."θ (deg)"=153.0, enum."Re(offset)"=0.0, enum."Im(offset)"=0.0, enum."στ1"=0.0, enum."στS"=0.0, enum."στN"=0.0, enum."τ11"=0.0, enum."τ12"=0.0, enum."τ22"=0.0, enum."τN1"=0.0, enum."τN2"=0.0, enum."σηlogτ1"=0.0, enum."σηlogτS"=0.0, enum."σηlogτN"=0.0, enum."σlogτ1"=0.0, enum."σlogτS"=0.0, enum."σlogτN"=0.0, enum."σητ1"=0.0, enum."σητS"=0.0, enum."σητN"=0.0, enum."noiseT"=0.0, enum."plain"=23.0, enum."vproj"=-0.625}, "009_042224"={enum."ζ"=0.0, enum."τ1"=0.0, enum."τS"=0.0, enum."τN"=0.0, enum."τC"=0.0, enum."κ0"=0.0, enum."m1"=0.0, enum."m2"=0.0, enum."m3"=0.0, enum."T (K)"=4.0, enum."B (T)"=60.0, enum."θ (deg)"=53.0, enum."Re(offset)"=0.0, enum."Im(offset)"=0.0, enum."στ1"=0.0, enum."στS"=0.0, enum."στN"=0.0, enum."τ11"=0.0, enum."τ12"=0.0, enum."τ22"=0.0, enum."τN1"=0.0, enum."τN2"=0.0, enum."σηlogτ1"=0.0, enum."σηlogτS"=0.0, enum."σηlogτN"=0.0, enum."σlogτ1"=0.0, enum."σlogτS"=0.0, enum."σlogτN"=0.0, enum."σητ1"=0.0, enum."σητS"=0.0, enum."σητN"=0.0, enum."noiseT"=0.0, enum."plain"=23.0, enum."vproj"=0.415}, "010_040924"={enum."ζ"=0.0, enum."τ1"=0.0, enum."τS"=0.0, enum."τN"=0.0, enum."τC"=0.0, enum."κ0"=0.0, enum."m1"=0.0, enum."m2"=0.0, enum."m3"=0.0, enum."T (K)"=4.0, enum."B (T)"=60.0, enum."θ (deg)"=30.0, enum."Re(offset)"=0.0, enum."Im(offset)"=0.0, enum."στ1"=0.0, enum."στS"=0.0, enum."στN"=0.0, enum."τ11"=0.0, enum."τ12"=0.0, enum."τ22"=0.0, enum."τN1"=0.0, enum."τN2"=0.0, enum."σηlogτ1"=0.0, enum."σηlogτS"=0.0, enum."σηlogτN"=0.0, enum."σlogτ1"=0.0, enum."σlogτS"=0.0, enum."σlogτN"=0.0, enum."σητ1"=0.0, enum."σητS"=0.0, enum."σητN"=0.0, enum."noiseT"=0.0, enum."plain"=23.0, enum."vproj"=0.6}, "010_041024"={enum."ζ"=0.0, enum."τ1"=0.0, enum."τS"=0.0, enum."τN"=0.0, enum."τC"=0.0, enum."κ0"=0.0, enum."m1"=0.0, enum."m2"=0.0, enum."m3"=0.0, enum."T (K)"=4.0, enum."B (T)"=60.0, enum."θ (deg)"=95.0, enum."Re(offset)"=0.0, enum."Im(offset)"=0.0, enum."στ1"=0.0, enum."στS"=0.0, enum."στN"=0.0, enum."τ11"=0.0, enum."τ12"=0.0, enum."τ22"=0.0, enum."τN1"=0.0, enum."τN2"=0.0, enum."σηlogτ1"=0.0, enum."σηlogτS"=0.0, enum."σηlogτN"=0.0, enum."σlogτ1"=0.0, enum."σlogτS"=0.0, enum."σlogτN"=0.0, enum."σητ1"=0.0, enum."σητS"=0.0, enum."σητN"=0.0, enum."noiseT"=0.0, enum."plain"=23.0, enum."vproj"=-0.057}, "010_041124"={enum."ζ"=0.0, enum."τ1"=0.0, enum."τS"=0.0, enum."τN"=0.0, enum."τC"=0.0, enum."κ0"=0.0, enum."m1"=0.0, enum."m2"=0.0, enum."m3"=0.0, enum."T (K)"=4.0, enum."B (T)"=60.0, enum."θ (deg)"=151.0, enum."Re(offset)"=0.0, enum."Im(offset)"=0.0, enum."στ1"=0.0, enum."στS"=0.0, enum."στN"=0.0, enum."τ11"=0.0, enum."τ12"=0.0, enum."τ22"=0.0, enum."τN1"=0.0, enum."τN2"=0.0, enum."σηlogτ1"=0.0, enum."σηlogτS"=0.0, enum."σηlogτN"=0.0, enum."σlogτ1"=0.0, enum."σlogτS"=0.0, enum."σlogτN"=0.0, enum."σητ1"=0.0, enum."σητS"=0.0, enum."σητN"=0.0, enum."noiseT"=0.0, enum."plain"=23.0, enum."vproj"=-0.615}, "010_042224"={enum."ζ"=0.0, enum."τ1"=0.0, enum."τS"=0.0, enum."τN"=0.0, enum."τC"=0.0, enum."κ0"=0.0, enum."m1"=0.0, enum."m2"=0.0, enum."m3"=0.0, enum."T (K)"=4.0, enum."B (T)"=60.0, enum."θ (deg)"=65.0, enum."Re(offset)"=0.0, enum."Im(offset)"=0.0, enum."στ1"=0.0, enum."στS"=0.0, enum."στN"=0.0, enum."τ11"=0.0, enum."τ12"=0.0, enum."τ22"=0.0, enum."τN1"=0.0, enum."τN2"=0.0, enum."σηlogτ1"=0.0, enum."σηlogτS"=0.0, enum."σηlogτN"=0.0, enum."σlogτ1"=0.0, enum."σlogτS"=0.0, enum."σlogτN"=0.0, enum."σητ1"=0.0, enum."σητS"=0.0, enum."σητN"=0.0, enum."noiseT"=0.0, enum."plain"=23.0, enum."vproj"=0.288}, "011_040924"={enum."ζ"=0.0, enum."τ1"=0.0, enum."τS"=0.0, enum."τN"=0.0, enum."τC"=0.0, enum."κ0"=0.0, enum."m1"=0.0, enum."m2"=0.0, enum."m3"=0.0, enum."T (K)"=4.0, enum."B (T)"=60.0, enum."θ (deg)"=60.0, enum."Re(offset)"=0.0, enum."Im(offset)"=0.0, enum."στ1"=0.0, enum."στS"=0.0, enum."στN"=0.0, enum."τ11"=0.0, enum."τ12"=0.0, enum."τ22"=0.0, enum."τN1"=0.0, enum."τN2"=0.0, enum."σηlogτ1"=0.0, enum."σηlogτS"=0.0, enum."σηlogτN"=0.0, enum."σlogτ1"=0.0, enum."σlogτS"=0.0, enum."σlogτN"=0.0, enum."σητ1"=0.0, enum."σητS"=0.0, enum."σητN"=0.0, enum."noiseT"=0.0, enum."plain"=23.0, enum."vproj"=0.348}, "011_041024"={enum."ζ"=0.0, enum."τ1"=0.0, enum."τS"=0.0, enum."τN"=0.0, enum."τC"=0.0, enum."κ0"=0.0, enum."m1"=0.0, enum."m2"=0.0, enum."m3"=0.0, enum."T (K)"=4.0, enum."B (T)"=60.0, enum."θ (deg)"=85.0, enum."Re(offset)"=0.0, enum."Im(offset)"=0.0, enum."στ1"=0.0, enum."στS"=0.0, enum."στN"=0.0, enum."τ11"=0.0, enum."τ12"=0.0, enum."τ22"=0.0, enum."τN1"=0.0, enum."τN2"=0.0, enum."σηlogτ1"=0.0, enum."σηlogτS"=0.0, enum."σηlogτN"=0.0, enum."σlogτ1"=0.0, enum."σlogτS"=0.0, enum."σlogτN"=0.0, enum."σητ1"=0.0, enum."σητS"=0.0, enum."σητN"=0.0, enum."noiseT"=0.0, enum."plain"=23.0, enum."vproj"=0.065}, "011_041124"={enum."ζ"=0.0, enum."τ1"=0.0, enum."τS"=0.0, enum."τN"=0.0, enum."τC"=0.0, enum."κ0"=0.0, enum."m1"=0.0, enum."m2"=0.0, enum."m3"=0.0, enum."T (K)"=4.0, enum."B (T)"=60.0, enum."θ (deg)"=157.0, enum."Re(offset)"=0.0, enum."Im(offset)"=0.0, enum."στ1"=0.0, enum."στS"=0.0, enum."στN"=0.0, enum."τ11"=0.0, enum."τ12"=0.0, enum."τ22"=0.0, enum."τN1"=0.0, enum."τN2"=0.0, enum."σηlogτ1"=0.0, enum."σηlogτS"=0.0, enum."σηlogτN"=0.0, enum."σlogτ1"=0.0, enum."σlogτS"=0.0, enum."σlogτN"=0.0, enum."σητ1"=0.0, enum."σητS"=0.0, enum."σητN"=0.0, enum."noiseT"=0.0, enum."plain"=23.0, enum."vproj"=-0.648}, "011_042224"={enum."ζ"=0.0, enum."τ1"=0.0, enum."τS"=0.0, enum."τN"=0.0, enum."τC"=0.0, enum."κ0"=0.0, enum."m1"=0.0, enum."m2"=0.0, enum."m3"=0.0, enum."T (K)"=4.0, enum."B (T)"=60.0, enum."θ (deg)"=160.0, enum."Re(offset)"=0.0, enum."Im(offset)"=0.0, enum."στ1"=0.0, enum."στS"=0.0, enum."στN"=0.0, enum."τ11"=0.0, enum."τ12"=0.0, enum."τ22"=0.0, enum."τN1"=0.0, enum."τN2"=0.0, enum."σηlogτ1"=0.0, enum."σηlogτS"=0.0, enum."σηlogτN"=0.0, enum."σlogτ1"=0.0, enum."σlogτS"=0.0, enum."σlogτN"=0.0, enum."σητ1"=0.0, enum."σητS"=0.0, enum."σητN"=0.0, enum."noiseT"=0.0, enum."plain"=23.0, enum."vproj"=-0.661}, "012_041024"={enum."ζ"=0.0, enum."τ1"=0.0, enum."τS"=0.0, enum."τN"=0.0, enum."τC"=0.0, enum."κ0"=0.0, enum."m1"=0.0, enum."m2"=0.0, enum."m3"=0.0, enum."T (K)"=4.0, enum."B (T)"=60.0, enum."θ (deg)"=75.0, enum."Re(offset)"=0.0, enum."Im(offset)"=0.0, enum."στ1"=0.0, enum."στS"=0.0, enum."στN"=0.0, enum."τ11"=0.0, enum."τ12"=0.0, enum."τ22"=0.0, enum."τN1"=0.0, enum."τN2"=0.0, enum."σηlogτ1"=0.0, enum."σηlogτS"=0.0, enum."σηlogτN"=0.0, enum."σlogτ1"=0.0, enum."σlogτS"=0.0, enum."σlogτN"=0.0, enum."σητ1"=0.0, enum."σητS"=0.0, enum."σητN"=0.0, enum."noiseT"=0.0, enum."plain"=23.0, enum."vproj"=0.183}, "013_041024"={enum."ζ"=0.0, enum."τ1"=0.0, enum."τS"=0.0, enum."τN"=0.0, enum."τC"=0.0, enum."κ0"=0.0, enum."m1"=0.0, enum."m2"=0.0, enum."m3"=0.0, enum."T (K)"=4.0, enum."B (T)"=60.0, enum."θ (deg)"=45.0, enum."Re(offset)"=0.0, enum."Im(offset)"=0.0, enum."στ1"=0.0, enum."στS"=0.0, enum."στN"=0.0, enum."τ11"=0.0, enum."τ12"=0.0, enum."τ22"=0.0, enum."τN1"=0.0, enum."τN2"=0.0, enum."σηlogτ1"=0.0, enum."σηlogτS"=0.0, enum."σηlogτN"=0.0, enum."σlogτ1"=0.0, enum."σlogτS"=0.0, enum."σlogτN"=0.0, enum."σητ1"=0.0, enum."σητS"=0.0, enum."σητN"=0.0, enum."noiseT"=0.0, enum."plain"=23.0, enum."vproj"=0.494}, "013_042224"={enum."ζ"=0.0, enum."τ1"=0.0, enum."τS"=0.0, enum."τN"=0.0, enum."τC"=0.0, enum."κ0"=0.0, enum."m1"=0.0, enum."m2"=0.0, enum."m3"=0.0, enum."T (K)"=4.0, enum."B (T)"=60.0, enum."θ (deg)"=163.0, enum."Re(offset)"=0.0, enum."Im(offset)"=0.0, enum."στ1"=0.0, enum."στS"=0.0, enum."στN"=0.0, enum."τ11"=0.0, enum."τ12"=0.0, enum."τ22"=0.0, enum."τN1"=0.0, enum."τN2"=0.0, enum."σηlogτ1"=0.0, enum."σηlogτS"=0.0, enum."σηlogτN"=0.0, enum."σlogτ1"=0.0, enum."σlogτS"=0.0, enum."σlogτN"=0.0, enum."σητ1"=0.0, enum."σητS"=0.0, enum."σητN"=0.0, enum."noiseT"=0.0, enum."plain"=23.0, enum."vproj"=-0.674}}, 10 "all full filenames":map{string, path}(c390), 15 "what? OUT":T1={"ignore set of !"=TRUE, "set (1T|2B)"=0, "ignore θ !"=FALSE, "ignore B !"=FALSE, "T (K)"=1.0, "ignore T !"=TRUE, "θ (∘)"=0.0, "B (T)"=0.0, "lookup"={"set of lookup"={0=1.0, 1=2.0}, "all set of"={}, "T lookup"={0=0.12, 1=0.122, 2=0.14, 3=0.148, 4=0.15, 5=0.157, 6=0.16, 7=0.168, 8=0.17, 9=0.178, 10=0.179, 11=0.18, 12=0.19, 13=0.197, 14=0.2, 15=0.249, 16=0.25, 17=0.255, 18=0.26, 19=0.3, 20=0.307, 21=0.308, 22=0.31, 23=0.36, 24=0.42, 25=0.43, 26=0.438, 27=0.512, 28=0.52, 29=0.53, 30=0.61, 31=0.62, 32=0.63, 33=0.677, 34=0.81, 35=0.82, 36=0.83, 37=1.0, 38=1.1, 39=1.12, 40=1.13, 41=1.25, 42=1.28, 43=1.31, 44=1.39, 45=1.5, 46=1.52, 47=1.55, 48=1.6, 49=1.7, 50=1.8, 51=1.9, 52=2.1, 53=2.3, 54=3.0, 55=3.07, 56=3.1, 57=3.11, 58=5.5, 59=5.7, 60=5.75}, "θ lookup"={0=0.0, 1=30.0, 2=45.0, 3=60.0, 4=90.0}, "B lookup"={0=0.0, 1=1.0, 2=2.0, 3=4.0, 4=5.0, 5=6.0, 6=7.0, 7=8.0, 8=9.0, 9=10.0, 10=11.0, 11=12.0}, "all T's"={}, "all θ's"={}, "all B's"={}, "all sides"={4000.0, 8000.0}, "side lookup"={0=4000.0, 1=8000.0}}} {"B (T)" items=["0.000", "1.000", "2.000", "4.000", "5.000", "6.000", "7.000", "8.000", "9.000", "10.000", "11.000", "12.000"]; "θ (∘)" items=["0.000", "30.000", "45.000", "60.000", "90.000"]; "T (K)" items=["0.120", "0.122", "0.140", "0.148", "0.150", "0.157", "0.160", "0.168", "0.170", "0.178", "0.179", "0.180", "0.190", "0.197", "0.200", "0.249", "0.250", "0.255", "0.260", "0.300", "0.307", "0.308", "0.310", "0.360", "0.420", "0.430", "0.438", "0.512", "0.520", "0.530", "0.610", "0.620", "0.630", "0.677", "0.810", "0.820", "0.830", "1.000", "1.100", "1.120", "1.130", "1.250", "1.280", "1.310", "1.390", "1.500", "1.520", "1.550", "1.600", "1.700", "1.800", "1.900", "2.100", "2.300", "3.000", "3.070", "3.100", "3.110", "5.500", "5.700", "5.750"]; "set (1T|2B)" items=["1", "2"]})   [LabVIEW 2021]
uses:
  3-lorentzian-parameters.ctl
  filename-action.ctl
  3-lorentzian-heat-response action.ctl
  <vilib>/Utility/miscctls.llb/LVMapReplaceAction.ctl
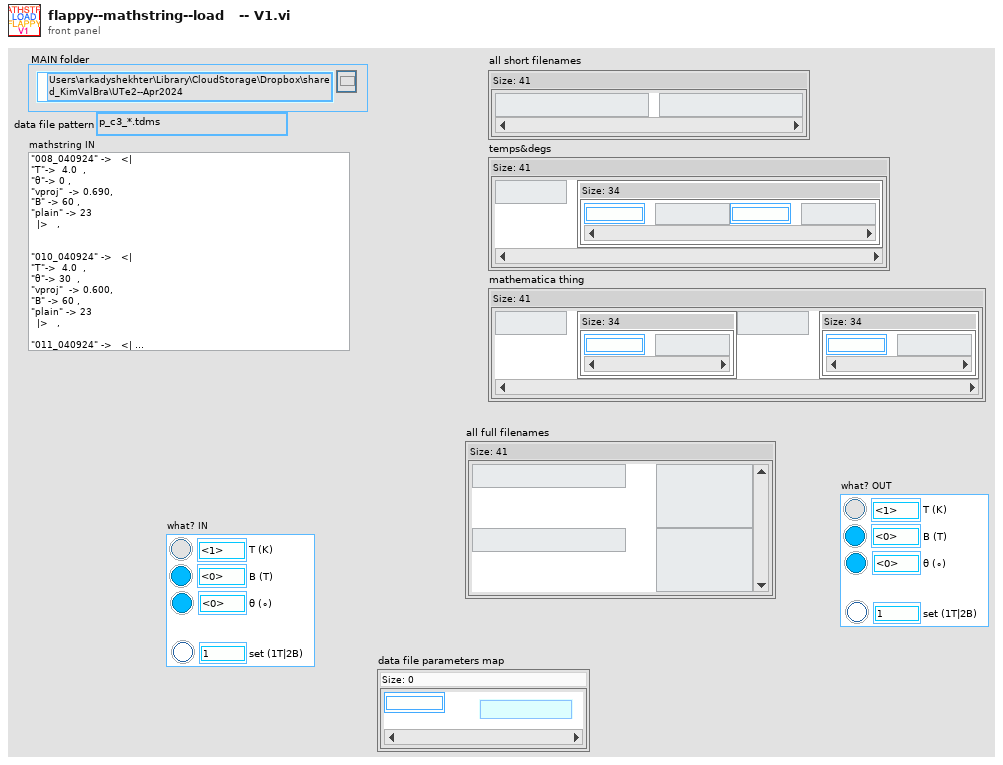
[diagram p1: front panel]
types:
  T1 = cluster{"ignore set of !":bool, "set (1T|2B)":i32, "ignore θ !":bool, "ignore B !":bool, "T (K)":dbl, "ignore T !":bool, "θ (∘)":dbl, "B (T)":dbl, "lookup":cluster{"set of lookup":map{i32, dbl}, "all set of":set{dbl}, "T lookup":map{i32, dbl}, "θ lookup":map{i32, dbl}, "B lookup":map{i32, dbl}, "all T's":set{dbl}, "all θ's":set{dbl}, "all B's":set{dbl}, "all sides":set{dbl}, "side lookup":map{i32, dbl}}}
  T2 = typedef "3-lorentzian-parameters.ctl" = enum16{"ζ", "τ1", "τS", "τN", "τC", "κ0", "m1", "m2", "m3", "T (K)", "B (T)", "θ (deg)", "side (S|R)", "set of (B|T)", "Re(offset)", "Im(offset)", "στ1", "στ1-", "στ1+", "στS", "στS-", "στS+", "στN", "στN-", "στN+", "τ11", "τ12", "τ21", "τ22", "τN1", "τN2", "σηlogτ1", "σηlogτS", "σηlogτN", "σlogτ1", "σlogτS", "σlogτN", "σητ1", "σητS", "σητN", "noiseT", "plain", "vproj"}
  T3 = typedef "filename-action.ctl" = enum16{"rewrite", "parse", "force pattern", "uniquenum", "get T", "get B", "get ind", "get deg", "get name", "get folder", "get extension", "get basename", "get side", "get setof", "getID", "getIDStock", "remove prefix", "get36thing", "getplain", "getvproj"}
  T4 = typedef "3-lorentzian-heat-response action.ctl" = enum16{"calc R", "create string", "calc m1m2m3", "dζ", "dT1", "dτS", "dτN", "dτC", "d-all", "dκ0", "T(K)", "m1", "m2", "m3", "parse string", "θ (deg)", "B (T)", "onlygrads", "newton", "create emty string", "simple2nd", "calc R2", "ScalarProd", "ScalarProd-diff", "nothing", "ScalarProd-eta", "tolog", "ignore", "three2nd", "eta-errors"}
  T5 = typedef "LVMapReplaceAction.ctl" = enum32{"Modify Entry only if found", "Add or Modify Entry", "Delete Entry"}
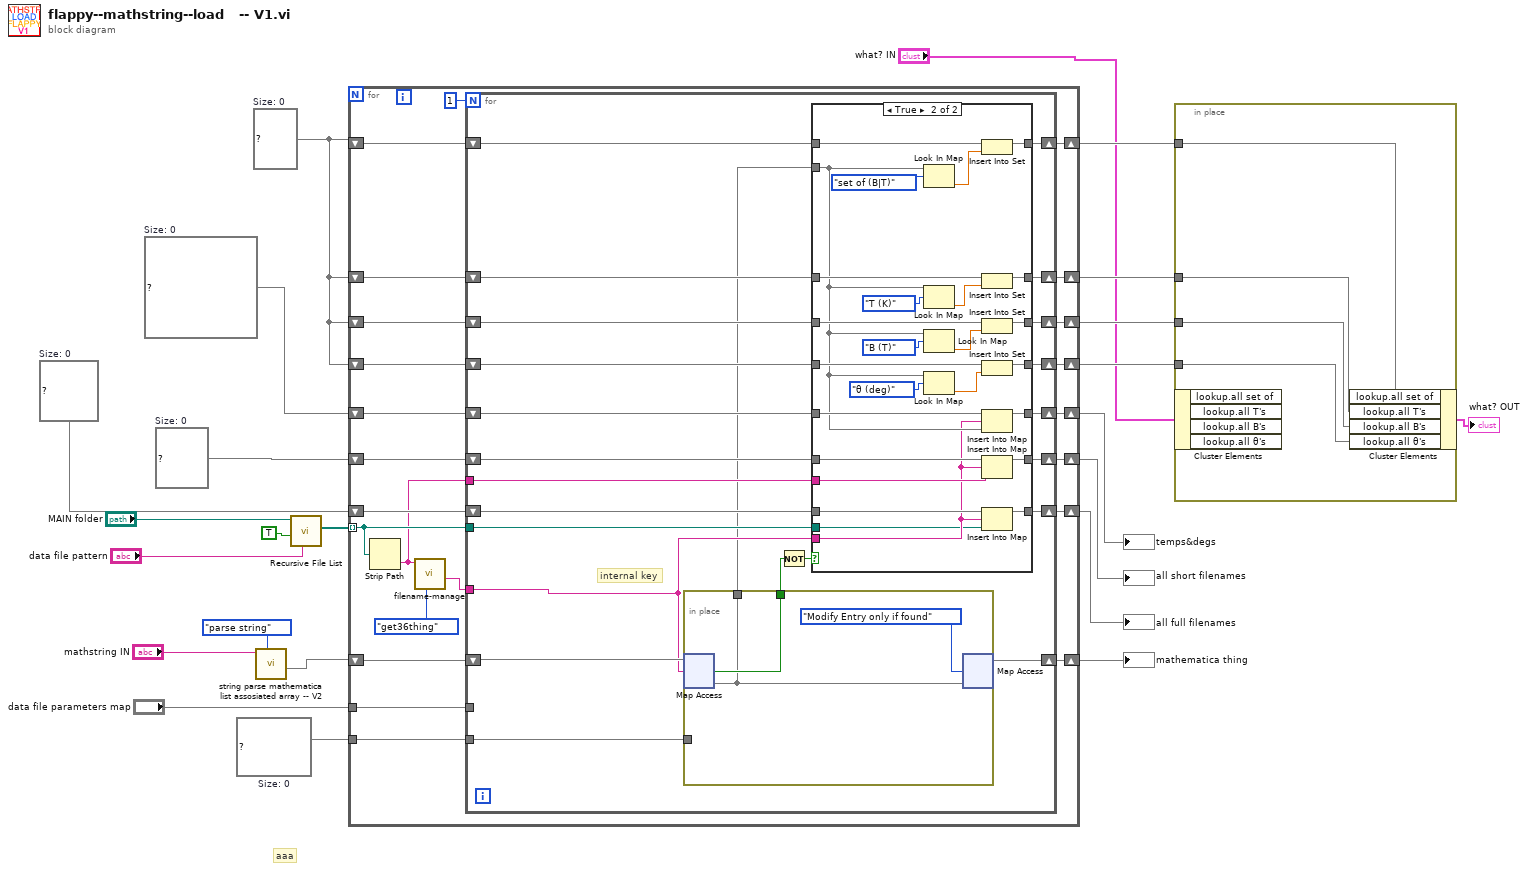
[diagram p0: block diagram]
diagram:
  w14 = map{string, path} {}  # Size: 0
  w22 = map{T2, dbl} {}  # Size: 0
  w21 = set{dbl} {}  # Size: 0
  w23 = map{string, map{T2, dbl}} {}  # Size: 0
  w18 = map{string, string} {}  # Size: 0
  # "aaa"
  n1 = call "string parse mathematica list assosiated array -- V2.vi"("action"=3-lorentzian-heat-response_action."parse string" ("derivative"), "string IN"="mathstring IN") -> ("actually found Map OUT"=w1:map{string, map{T2, dbl}})  [unwired: 6 in, 3 out]
  n2 = call <vilib>:"Recursive File List.vi"("pattern"="data file pattern", "Continue Recursing on Error? (F)"=TRUE, "Folder Path"="MAIN folder") -> ("All Files in Dir"=w15:path[])  [unwired: 4 in, 4 out]
  n3 = for {
    tunnel: w15 -> [w26] mode=indexing
    shift-right: [w36] -> w8
    shift-left: w1 -> [w45]
    shift-right: [w33] -> w20
    shift-left: w18 -> [w44]
    shift-right: [w32] -> w19
    shift-left: w23 -> [w40]
    shift-right: [w42] -> w12
    shift-left: w21 -> [w35]
    shift-right: [w34] -> w11
    shift-left: w21 -> [w43]
    tunnel: w22 -> [w39]
    shift-right: [w30] -> w10
    shift-left: w21 -> [w41]
    tunnel: "data file parameters map" -> [w38]
    shift-right: [w31] -> w13
    shift-left: w21 -> [w37]
    shift-right: [w27] -> w17
    shift-left: w14 -> [w28]
    n4 = Strip Path(path=w26) -> (name=w25:string)  [unwired: 1 out]
    n5 = call "filename-manage.vi"("filename-action"=filename-action."get36thing", "file name IN"=w25) -> ("string OUT"=w29:string)  [unwired: 7 in, 2 out]
    n6 = for {
      N: 1 -> [_]
      tunnel: w38 -> [_]
      tunnel: w25 -> [w51]
      tunnel: w29 -> [w49]
      shift-right: [w60] -> w36
      shift-left: w45 -> [w69]
      shift-right: [w64] -> w42
      shift-left: w35 -> [w59]
      shift-right: [w58] -> w34
      shift-left: w43 -> [w65]
      shift-right: [w54] -> w30
      shift-left: w41 -> [w63]
      shift-right: [w55] -> w31
      shift-left: w37 -> [w61]
      shift-right: [w56] -> w32
      shift-left: w40 -> [w62]
      shift-right: [w57] -> w33
      shift-left: w44 -> [w68]
      tunnel: w39 -> [w48]
      shift-right: [w52] -> w27
      shift-left: w28 -> [w53]
      tunnel: w26 -> [w50]
      # "internal key"
      n7 = in-place {
        in-place-border: [w104] -> w67
        in-place-border: w48 -> [_]
        in-place-border: [w103] -> w47
        n8 = in-place-map #1(w69, w49) -> (w103:map{T2, dbl}, w104:bool)  [unwired: 1 in]
        n9 = in-place-map #1(w103, LVMapReplaceAction."Modify Entry only if found" ("action")) -> (w60:map{string, map{T2, dbl}})  [unwired: 2 out]
      }
      n10 = Not(x=w67) -> (.not. x?=w66:bool)
      n11 = case shown="True" w66 {
        tunnel: w68 -> [w76 w102]
        tunnel: [w76 w101] -> w57
        tunnel: w51 -> [_ w100]
        tunnel: w49 -> [_ w78]
        tunnel: w65 -> [w74 w99]
        tunnel: [w74 w98] -> w58
        tunnel: w59 -> [w75 w97]
        tunnel: [w75 w96] -> w64
        tunnel: [w72 w95] -> w54
        tunnel: w63 -> [w72 w94]
        tunnel: w47 -> [_ w83]
        tunnel: w62 -> [w73 w93]
        tunnel: [w73 w92] -> w56
        tunnel: [w71 w85] -> w55
        tunnel: w61 -> [w71 w84]
        tunnel: w53 -> [w70 w80]
        tunnel: [w70 w79] -> w52
        tunnel: w50 -> [_ w77]
        frame False {
        }
        frame True {
          n12 = Look In Map(map=w83, key=3-lorentzian-parameters."set of (B|T)") -> (value=w86:dbl)  [unwired: 1 in, 1 out]
          n13 = Look In Map(map=w83, key=3-lorentzian-parameters."T (K)") -> (value=w90:dbl)  [unwired: 1 in, 1 out]
          n14 = Look In Map(map=w83, key=3-lorentzian-parameters."B (T)") -> (value=w82:dbl)  [unwired: 1 in, 1 out]
          n15 = Look In Map(map=w83, key=3-lorentzian-parameters."θ (deg)") -> (value=w81:dbl)  [unwired: 1 in, 1 out]
          n16 = Insert Into Set(10:w86, 11:w84) -> (3:w85:set{dbl})  [unwired: 1 out]
          n17 = Insert Into Set(10:w90, 11:w94) -> (3:w95:set{dbl})  [unwired: 1 out]
          n18 = Insert Into Set(10:w82, 11:w99) -> (3:w98:set{dbl})  [unwired: 1 out]
          n19 = Insert Into Set(10:w81, 11:w97) -> (3:w96:set{dbl})  [unwired: 1 out]
          n20 = Insert Into Map(map in=w93, key=w78, value=w83) -> (map out=w92:map{string, map{T2, dbl}})  [unwired: 2 out]
          n21 = Insert Into Map(map in=w102, key=w78, value=w100) -> (map out=w101:map{string, string})  [unwired: 2 out]
          n22 = Insert Into Map(map in=w80, key=w78, value=w77) -> (map out=w79:map{string, path})  [unwired: 2 out]
        }
      }
    }
  }
  "all short filenames" <- w20
  "temps&degs" <- w19
  "mathematica thing" <- w8
  "all full filenames" <- w17
  n23 = in-place {
    in-place-border: w13 -> [w109]
    in-place-border: w12 -> [w106]
    in-place-border: w11 -> [w107]
    in-place-border: w10 -> [w108]
    n24 = in-place-cluster #2("what? IN") -> ()  [unwired: 4 out]
    n25 = in-place-cluster #2("lookup.all set of"=w109, "lookup.all T's"=w108, "lookup.all B's"=w107, "lookup.all θ's"=w106) -> (→"what? OUT":T1)
  }
